vi "Initialize SLSC Switch Custom Device.vi"(8 "error in (no error)":errorcluster, 11 "SLSC Custom Device Ref in":T1 format="%.0x") -> (0 "error out":errorcluster, 2 "Endpoint Configuration Section Ref":T1 format="%.0x", 3 "SLSC Custom Device  Ref out":T1 format="%.0x")   [LabVIEW 2017, in "SLSC Switch Scripting.lvlib"]
uses:
  SLSC Switch Scripting.lvlib
  <vilib>/NI Veristand/Custom Device API/Custom Device Item Ref.ctl
  SLSC Scripting Constants.vi
  <vilib>/NI Veristand/Custom Device API/Set Item Property (String).vi
  <vilib>/NI VeriStand/Custom Device API/Custom Device API.lvlib
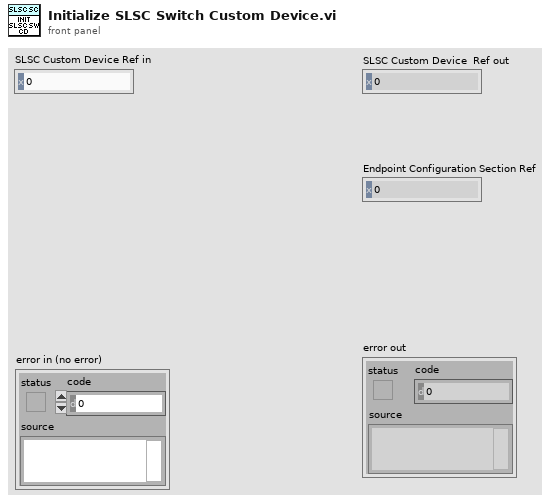
[diagram p1: front panel]
types:
  T1 = typedef "Custom Device API.lvlib/Custom Device Item Ref.ctl" = u64
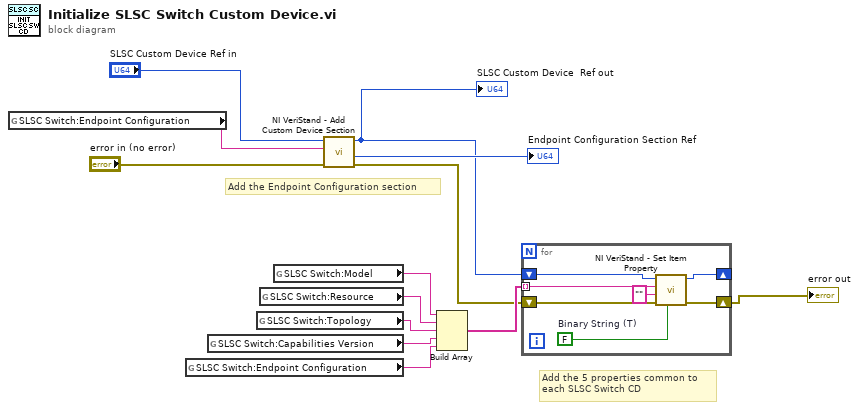
[diagram p0: block diagram]
diagram:
  # "Add the 5 properties common to\neach SLSC Switch CD"
  # "Add the Endpoint Configuration section"
  n1 = global read "SLSC Scripting Constants.vi" "SLSC Switch:Endpoint Configuration"() -> (w11:string)
  n2 = global read "SLSC Scripting Constants.vi" "SLSC Switch:Endpoint Configuration"() -> (w5:string)
  n3 = global read "SLSC Scripting Constants.vi" "SLSC Switch:Capabilities Version"() -> (w6:string)
  n4 = global read "SLSC Scripting Constants.vi" "SLSC Switch:Topology"() -> (w7:string)
  n5 = global read "SLSC Scripting Constants.vi" "SLSC Switch:Resource"() -> (w8:string)
  n6 = global read "SLSC Scripting Constants.vi" "SLSC Switch:Model"() -> (w9:string)
  n7 = call <vilib>:"NI VeriStand - Add Custom Device Section.vi"("error in (no error)"="error in (no error)", "Section Name"=w11, "Parent Ref in"="SLSC Custom Device Ref in") -> ("error out"=w3:errorcluster, "Section Ptr"=→"Endpoint Configuration Section Ref":T1, "Parent Ref out"=w2:T1)  [unwired: 5 in, 1 out]
  "SLSC Custom Device  Ref out" <- w2
  n8 = Build Array(w9, w8, w7, w6, w5) -> (w4:string[])
  n9 = for {
    tunnel: w4 -> [w18] mode=indexing
    shift-right: [w17] -> w1
    shift-left: w3 -> [w16]
    shift-right: [w15] -> _
    shift-left: w2 -> [w19]
    w20 = FALSE  # Binary String (T)
    n10 = call-poly <vilib>:"NI VeriStand - Set Item Property.vi"("Binary String (T)"=w20, "error in (no error)"=w16, "Value"="", "Property Name"=w18, "Item Ref in"=w19) -> ("error out"=w17:errorcluster, "Item Ref out"=w15:T1)  [unwired: 4 in, 1 out]
  }
  "error out" <- w1
